vi "Register for Events.vi"(8 "error in (no error)":errorcluster, 11 "BetterSearch in":refnum<class "BetterSearch.lvclass">) -> (0 "error out":errorcluster, 3 "BetterSearch out":refnum<class "BetterSearch.lvclass">)   [LabVIEW 2020, in "Better Search.lvlib" / "BetterSearch.lvclass"]
uses:
  BetterSearch.lvclass
  BetterSearch.lvclass/BetterSearch.ctl
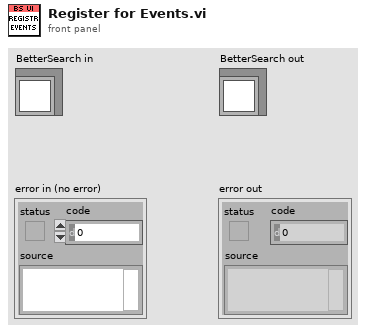
[diagram p1: front panel]
types:
  T1 = typedef "Better Search.lvlib/BetterSearch.lvclass/Edit Events.ctl" = cluster{"New Edit":refnum<user-event>, "Close Edit Panel":refnum<user-event>}
  T2 = typedef "Better Search.lvlib/BetterSearch.lvclass/Results Events.ctl" = cluster{"Close Results Panel":refnum<user-event>, "Show Search":refnum<user-event>, "Show Result":refnum<user-event>, "Progress WD":refnum<user-event>}
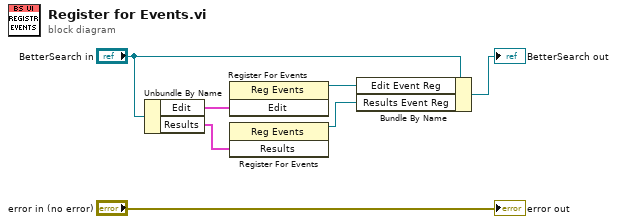
[diagram p0: block diagram]
diagram:
  n1 = Unbundle By Name("BetterSearch in") -> ("Edit"=w6:T1, "Results"=w2:T2)
  n2 = register-events(w6) -> (reference out=w5:refnum<event-registration>)  [unwired: 2 in, 1 out]
  n3 = register-events(w2) -> (reference out=w1:refnum<event-registration>)  [unwired: 2 in, 1 out]
  n4 = Bundle By Name(cluster="BetterSearch in", "Edit Event Reg"=w5, "Results Event Reg"=w1) -> (→"BetterSearch out":refnum<class "BetterSearch.lvclass">)
  "error out" <- "error in (no error)"
